vi "ROI entry-Obtain previous ROI file path.vi"() -> (0 "error out":errorcluster, 3 "Experiment folder path containing last ROI file":path)   [LabVIEW 2020]
panel:
  in  "error in":errorcluster
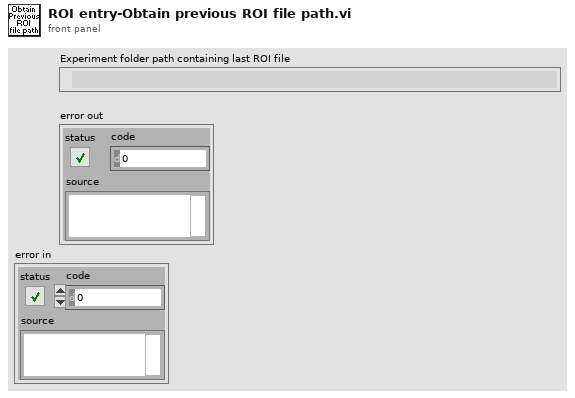
[diagram p1: front panel]
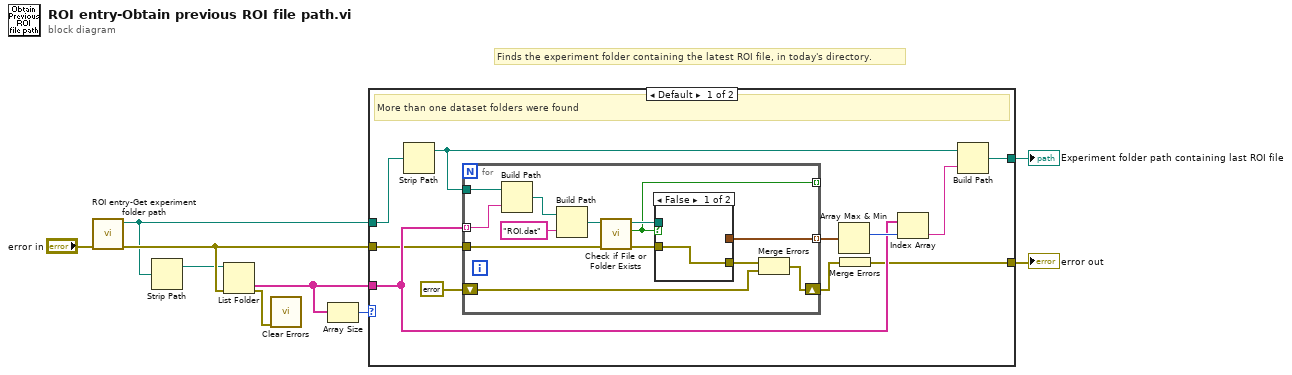
[diagram p0: block diagram]
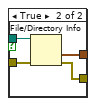
[diagram p2: hidden frame]
diagram:
  # "Finds the experiment folder containing the latest ROI file, in today's directory."
  n1 = call "ROI entry-Get experiment folder path.vi"("error in (no error)"="error in") -> ("error out"=w4:errorcluster, "Experiment folder path"=w2:path)  [unwired: 9 in]
  n2 = Strip Path(path=w2) -> (stripped path=w3:path)  [unwired: 1 out]
  n3 = List Folder(path=w3, error in=w4) -> (folder names=w7:string[], error out=w6:errorcluster)  [unwired: 2 in, 2 out]
  n4 = call <vilib>:"Clear Errors.vi"("error in (no error)"=w6) -> ()  [unwired: 5 in, 2 out]
  n5 = Array Size(array=w7) -> (size(s)=w9:i32)
  n6 = case shown="Default" w9 {
    tunnel: [w17 w39] -> w8
    tunnel: w7 -> [w19 _]
    tunnel: [w12 w40] -> w5
    tunnel: w4 -> [w15 w40]
    tunnel: w2 -> [w11 w39]
    frame Default {
      # "More than one dataset folders were found"
      n7 = Strip Path(path=w11) -> (stripped path=w10:path)  [unwired: 1 out]
      n8 = for {
        tunnel: w10 -> [w33]
        tunnel: w19 -> [w32] mode=indexing
        tunnel: [w31] -> w13 mode=indexing
        tunnel: [w26] -> _ mode=indexing
        tunnel: w15 -> [w24]
        shift-right: [w23] -> w16
        shift-left: errorcluster {"status"=FALSE, "code"=0, "source"=""} ("error IO") -> [w21]
        n9 = Build Path(base path=w33, name or relative path=w32) -> (appended path=w28:path)
        n10 = Build Path(base path=w28, name or relative path="ROI.dat") -> (appended path=w29:path)
        n11 = call <vilib>:"Check if File or Folder Exists.vi"("error in (no error)"=w24, "path"=w29) -> ("error out"=w25:errorcluster, "file or folder exists?"=w26:bool, "dup path"=w27:path)  [unwired: 7 in]
        n12 = case shown="False" w26 {
          tunnel: [_ w38] -> w31
          tunnel: w27 -> [_ w37]
          tunnel: w25 -> [w34 w36]
          tunnel: [w34 w35] -> w22
          frame False {
          }
          frame True {
            n13 = File/Directory Info(path=w37, error in=w36) -> (last mod=w38:timestamp, error out=w35:errorcluster)  [unwired: 5 out]
          }
        }
        n14 = Merge Errors(w22, w21) -> (w23:errorcluster)
      }
      n15 = Array Max & Min(array=w13) -> (max index (indices)=w20:i32)  [unwired: 3 out]
      n16 = Merge Errors(w16) -> (w12:errorcluster)
      n17 = Index Array(array=w19, index=w20) -> (element=w18:string)
      n18 = Build Path(base path=w10, name or relative path=w18) -> (appended path=w17:path)
    }
    frame 0, 1 {
      # "The daily directory contains just a single dataset folder (or none at all / fail-safe)"
    }
  }
  "error out" <- w5
  "Experiment folder path containing last ROI file" <- w8
